vi "S2C_FORNAX_Proc_LogDdsMsg.vi"(7 "Direction":enum16{"TX", "RX"}(ring), 8 "Error In":errorcluster, 11 "Msg In":string) -> (0 "Error Out":errorcluster, 3 "Msg Out":string)   [LabVIEW 2015]
doc: "Extracts the Viper message from the DDS data stream."
uses:
  S2C_FORNAX_Proc_Globals.vi
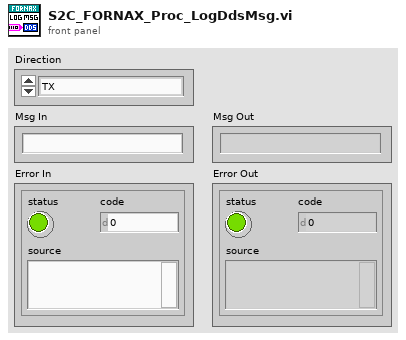
[diagram p1: front panel]
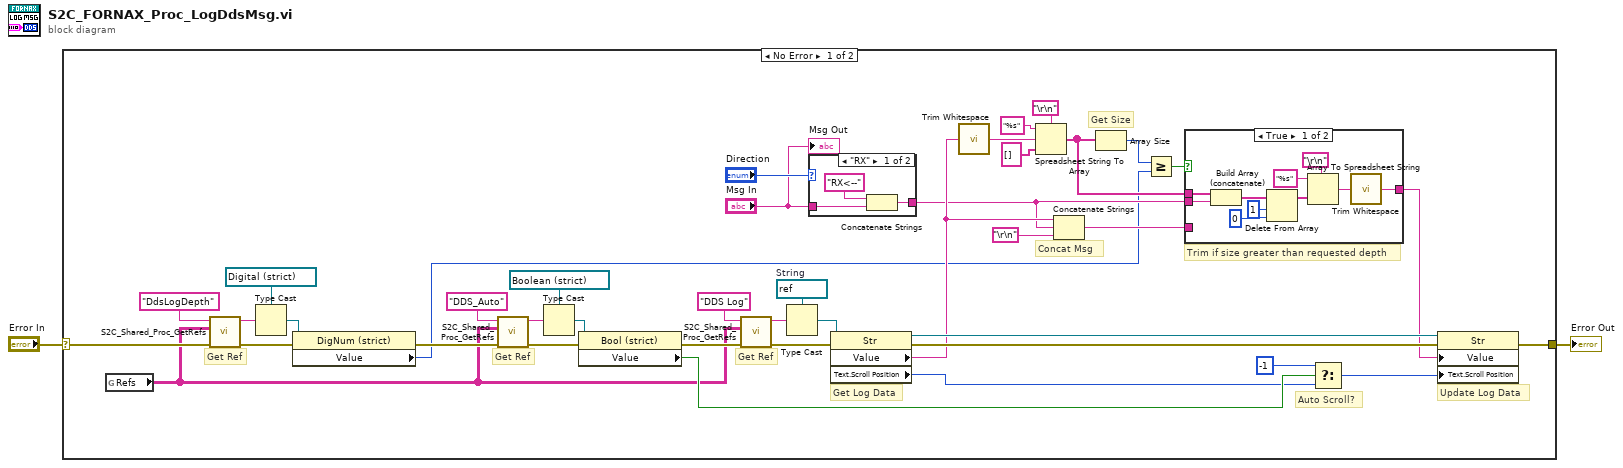
[diagram p0: block diagram]
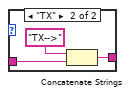
[diagram p2: hidden frame]
diagram:
  n1 = case shown="No Error" "Error In" {
    selector: "Error In" -> [w9 w61]
    tunnel: [w35 w61] -> w1
    frame No Error {
      w41 = refnum<vi> refnum  # String
      # "Get Ref"
      # "Trim if size greater than requested depth"
      # "Get Size"
      # "Concat Msg"
      # "Auto Scroll?"
      # "Get Ref"
      # "Update Log Data"
      # "Get Log Data"
      # "Get Ref"
      n2 = global read "S2C_FORNAX_Proc_Globals.vi" "Refs"() -> (w3:string[][])
      n3 = call "S2C_Shared_Proc_GetRefs.vi"("Error In"=w9, "Refs"=w3, "Label"="DdsLogDepth") -> ("Error Out"=w18:errorcluster, "Reference"=w17:string)  [unwired: 7 in]
      n4 = Type Cast(type=refnum<vi> refnum ("Numeric Control"), x=w17) -> (*(type *) &x=w16:refnum<vi>)
      n5 = property class="DigNum (strict)"(reference=w16, error in=w18) -> (error out=w13:errorcluster, "Value"=w4:i32)  [unwired: 1 out]
      n6 = call "S2C_Shared_Proc_GetRefs.vi"("Error In"=w13, "Refs"=w3, "Label"="DDS_Auto") -> ("Error Out"=w31:errorcluster, "Reference"=w32:string)  [unwired: 7 in]
      n7 = Type Cast(type=refnum<vi> refnum ("Boolean"), x=w32) -> (*(type *) &x=w33:refnum<vi>)
      n8 = property class="Bool (strict)"(reference=w33, error in=w31) -> (error out=w29:errorcluster, "Value"=w20:bool)  [unwired: 1 out]
      n9 = call "S2C_Shared_Proc_GetRefs.vi"("Error In"=w29, "Refs"=w3, "Label"="DDS Log") -> ("Error Out"=w42:errorcluster, "Reference"=w40:string)  [unwired: 7 in]
      n10 = Type Cast(type=w41, x=w40) -> (*(type *) &x=w39:refnum<vi>)
      n11 = case shown="\"RX\"" "Direction" {
        tunnel: "Msg In" -> [w46 w49]
        tunnel: [w44 w47] -> w6
        frame "RX" {
          n12 = Concatenate Strings("RX<--" ("string"), w46) -> (w44:string)
        }
        frame "TX" {
          n13 = Concatenate Strings("TX-->" ("string"), w49) -> (w47:string)
        }
      }
      n14 = property class="Str"(reference=w39, error in=w42) -> (reference out=w34:refnum<vi>, error out=w38:errorcluster, "Value"=w21:string, "Text.Scroll Position"=w10:u32)
      n15 = call <vilib>:"Trim Whitespace.vi"("string"=w21) -> ("trimmed string"=w8:string)  [unwired: 1 in]
      n16 = Spreadsheet String To Array(delimiter (Tab)="\r\n", format string="%s", spreadsheet string=w8, array type (2D Dbl)=string[] []) -> (array=w25:string[])
      n17 = Concatenate Strings(w21, w6, "\r\n") -> (w26:string)
      n18 = Array Size(array=w25) -> (size(s)=w14:i32)
      n19 = Greater Or Equal?(x=w14, y=w4) -> (x >= y?=w12:bool)
      n20 = case shown="True" w12 {
        tunnel: w6 -> [w57 _]
        tunnel: w25 -> [w58 _]
        tunnel: w26 -> [_ w60]
        tunnel: [w50 w60] -> w11
        frame True {
          n21 = Build Array (concatenate)(w58, w57) -> (w56:string[])
          n22 = Delete From Array(array=w56, length=1, index=0) -> (array with subset deleted=w54:string[])  [unwired: 1 out]
          n23 = Array To Spreadsheet String(delimiter (Tab)="\r\n", array=w54, 3:"%s" ("format string")) -> (spreadsheet string=w51:string)
          n24 = call <vilib>:"Trim Whitespace.vi"("string"=w51) -> ("trimmed string"=w50:string)  [unwired: 1 in]
        }
        frame False {
        }
      }
      n25 = Select(t=-1, s=w20, f=w10) -> (s? t:f=w36:u32)
      n26 = property class="Str"(reference=w34, error in=w38, "Value"=w11, "Text.Scroll Position"=w36) -> (error out=w35:errorcluster)  [unwired: 1 out]
      "Msg Out" <- "Msg In"
    }
    frame Error {
    }
  }
  "Error Out" <- w1
